vi "Read_Class_database.vi"(8 "error in (no error)":errorcluster caption="entrée d'erreur (pas d'erreur)", 11 "Class Instrument Firebase Altyor en entrée":refnum<class "Class Instrument Database Altyor.lvclass">) -> (0 "error out":errorcluster caption="sortie d'erreur", 2 "Database Altyor":refnum<class "Database Altyor.lvclass">, 3 "Class Instrument Firebase Altyor en sortie":refnum<class "Class Instrument Database Altyor.lvclass">)   [LabVIEW 2020, in "Library Instrument & Equipement.lvlib" / "Library Instruments.lvlib" / "Class Instrument Database Altyor.lvclass"]
uses:
  Class Instrument Database Altyor.lvclass
  Database/Database Altyor/Database Altyor.lvclass
  Class Instrument Database Altyor.lvclass/Class Instrument Database Altyor.ctl
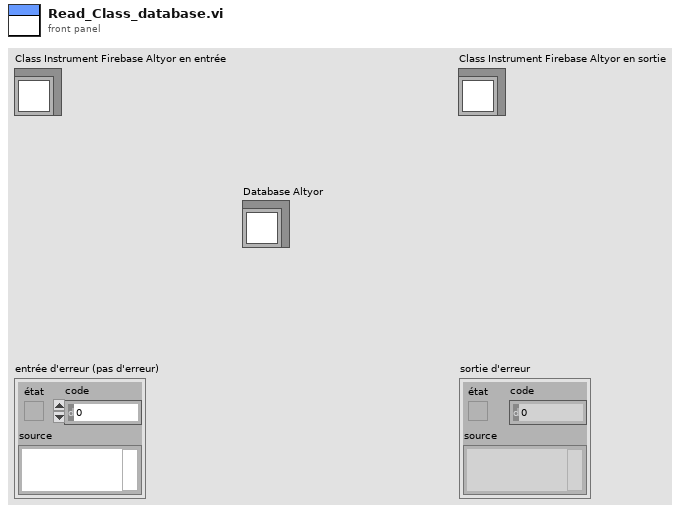
[diagram p1: front panel]
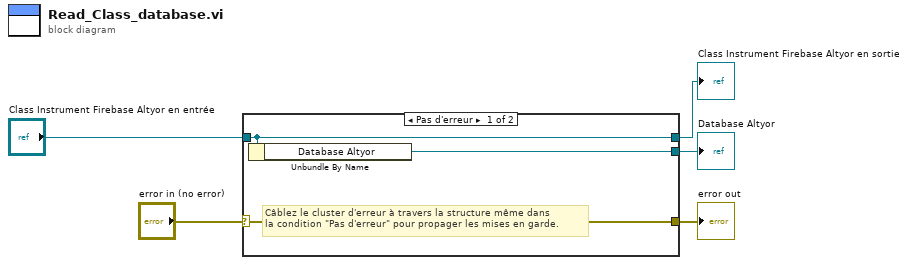
[diagram p0: block diagram]
diagram:
  n1 = case shown="Pas d'erreur" "error in (no error)" {
    selector: "error in (no error)" -> [w8 w10]
    tunnel: [w8 w10] -> w4
    tunnel: [w7 w9] -> w2
    tunnel: "Class Instrument Firebase Altyor en entrée" -> [w7 w9]
    tunnel: [w6 _] -> w1
    frame No Error {
      # "Câblez le cluster d'erreur à travers la structure même dans\nla condition \"Pas d'erreur\" pour propager les mises en garde."
      n2 = Unbundle By Name(w7) -> ("Database Altyor"=w6:refnum<class "Database Altyor.lvclass">)
    }
    frame Error {
    }
  }
  "error out" <- w4
  "Class Instrument Firebase Altyor en sortie" <- w2
  "Database Altyor" <- w1
